vi "Chi2_kernel.vi"(8 "error in":errorcluster caption="entrée d'erreur", 9 "Y":string[][](array[string]), 10 "X":string[][](array[string]), 11 "chi2_kernel":cluster{"gamma":dbl}={"gamma"=1.0}) -> (0 "error out":errorcluster caption="sortie d'erreur", 3 "Data":T1)   [LabVIEW 2020]
doc: "Computes the exponential chi-squared kernel X and Y.\n\nThe chi-squared kernel is computed between each pair of rows in X and Y. X and Y have to be non-negative. This kernel is most commonly applied to histograms.\n\nThe chi-squared kernel is given by :\n\nk(x, y) = exp(-gamma Sum [(x - y)^2 / (x + y)])\n\nIt can be interpreted as a weighted difference per entry.\n\nParameters : \n\n- X : array-like of shape (n_samples_X, n_features)\n\n- Y : array of shape (n_samples_Y, n_features)\n\n- gamma : float, default=1.\nScaling parameter of the chi2 kernel.\n\nReturns : \n\n- kernel_matrix : array of shape (n_samples_X, n_samples_Y)"
uses:
  Chi2_kernel.lvclass
panel:
  out "Chi2_kernel.lvclass":refnum<class "Chi2_kernel.lvclass">
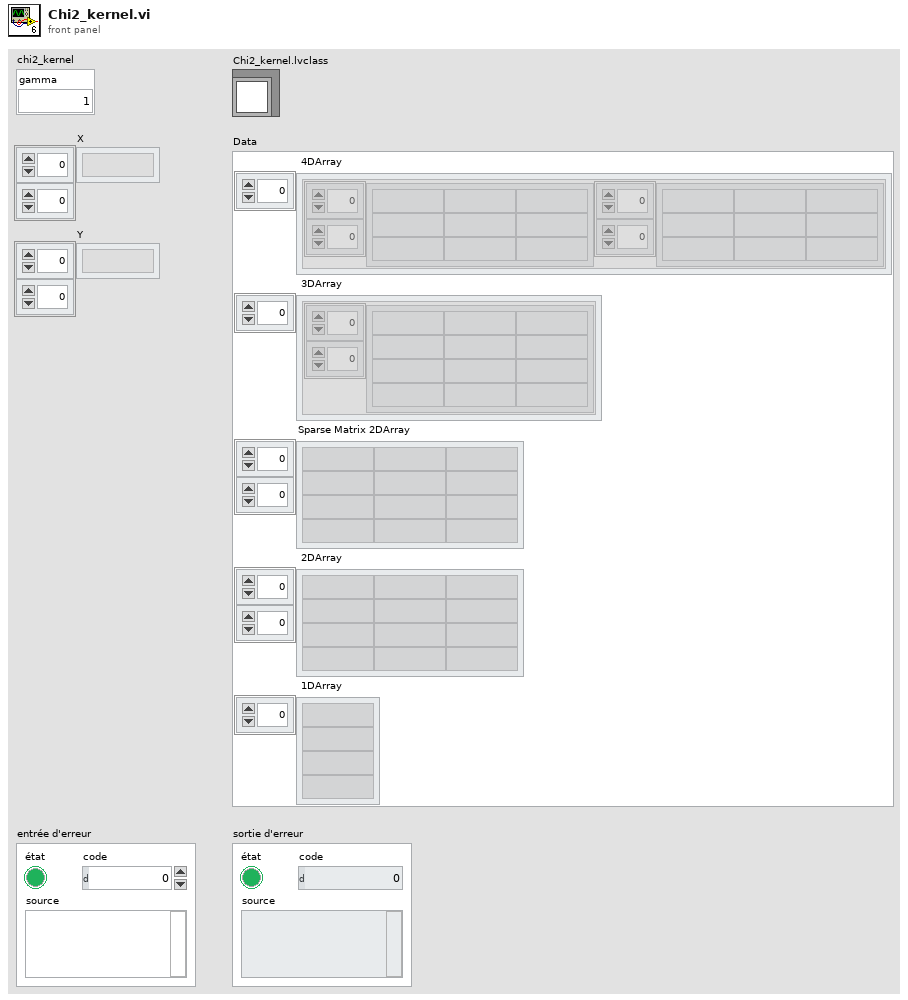
[diagram p1: front panel]
types:
  T1 = cluster{" 4DArray":cluster{"1":string[][], "2":string[][]}[], " 3DArray":cluster{"Tableau":string[][]}[], "Sparse Matrix 2DArray":string[][], " 2DArray":string[][], " 1DArray":string[]}
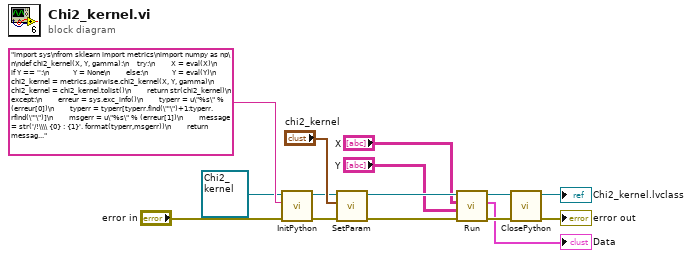
[diagram p0: block diagram]
diagram:
  n1 = call-dynamic "InitPython.vi"("error in (no error)"="error in", "Python Instruction"="import sys\nfrom sklearn import metrics\nimport numpy as np\n\ndef chi2_kernel(X, Y, gamma):\n    try:\n        X = eval(X)\n        if Y == '':\n            Y = None\n        else:\n            Y = eval(Y)\n        chi2_kernel = metrics.pairwise.chi2_kernel(X, Y, gamma)\n        chi2_kernel = chi2_kernel.tolist()\n        return str(chi2_kernel)\n    except:\n        erreur = sys.exc_info()\n        typerr = u\"%s\" % (erreur[0])\n        typerr = typerr[typerr.find(\"'\")+1:typerr.rfind(\"'\")]\n        msgerr = u\"%s\" % (erreur[1])\n        message = str('/!\\\\ {0} : {1}'. format(typerr,msgerr))\n        return message", "Scikit-learn en entrée"=refnum<class "Chi2_kernel.lvclass"> refnum ("Chi2_kernel.lvclass")) -> ("error out"=w12:errorcluster, "Scikit-learn en sortie"=w10:refnum<class "Chi2_kernel.lvclass">)  [unwired: 7 in]
  n2 = call-dynamic "SetParam.vi"("error in (no error)"=w12, "chi2_kernel"="chi2_kernel", "Chi2_kernel.lvclass"=w10) -> ("error out"=w8:errorcluster, "Chi2_kernel.lvclass"=w9:refnum<class "Chi2_kernel.lvclass">)  [unwired: 7 in]
  n3 = call-dynamic "Run.vi"("error in (no error)"=w8, "Y"="Y", "X"="X", "Chi2_kernel.lvclass"=w9) -> ("error out"=w6:errorcluster, "Data"=→"Data":T1, "Chi2_kernel.lvclass"=w7:refnum<class "Chi2_kernel.lvclass">)  [unwired: 5 in]
  n4 = call-dynamic "ClosePython.vi"("error in (no error)"=w6, "Scikit-learn en entrée"=w7) -> ("error out"=→"error out":errorcluster, "Scikit-learn en sortie"=→"Chi2_kernel.lvclass":refnum<class "Chi2_kernel.lvclass">)  [unwired: 8 in]
